vi "latch_lock.vi"(1 "Reset":bool, 2 "GO!":bool) -> (0 "ON":bool)   [LabVIEW 2012]
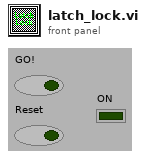
[diagram p1: front panel]
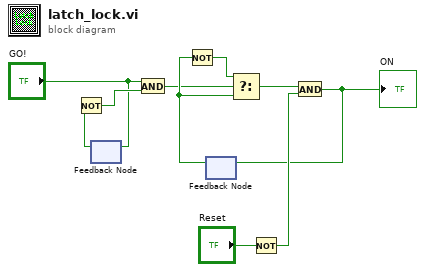
[diagram p0: block diagram]
diagram:
  n1 = feedback-in #1("GO!") -> ()
  n2 = feedback #1() -> (w7:bool)  [unwired: 1 out]
  n3 = Not(x=w7) -> (.not. x?=w4:bool)
  n4 = And(x="GO!", y=w4) -> (x .and. y?=w5:bool)
  n5 = feedback #2() -> (w10:bool)  [unwired: 1 out]
  n6 = Not(x=w10) -> (.not. x?=w6:bool)
  n7 = Select(t=w6, s=w5, f=w10) -> (s? t:f=w8:bool)
  n8 = Not(x="Reset") -> (.not. x?=w9:bool)
  n9 = And(x=w8, y=w9) -> (x .and. y?=w3:bool)
  "ON" <- w3
  n10 = feedback-in #2(w3) -> ()
